vi "Draw Horizontal Line.vi"(6 "Colour":u32(colorbox), 9 "Point 2":T1, 10 "Point 1":T1, 11 "Pixel Data in":u32[][](array[numeric])) -> (3 "Pixel Data out":u32[][](array[numeric]))   [LabVIEW 2022 SP3, in "Raster.lvlib"]
uses:
  Raster.lvlib
  Point 2D.ctl
  <vilib>/Utility/High Resolution Relative Seconds.vi
  Utility/Utility.lvlib
panel:
  out "Processing Time [s]":dbl format="%.1p"
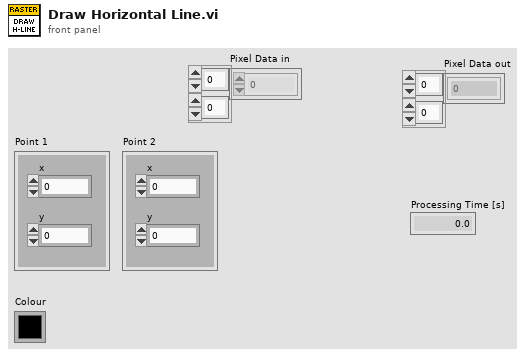
[diagram p1: front panel]
types:
  T1 = typedef "Raster.lvlib/Point 2D.ctl" = cluster{"x":i32, "y":i32}
  T2 = cluster{"pointer":u64, "size_0":u32, "stride_0":i32, "size_1":u32, "stride_1":i32, "element size":u32, "subarray?":bool}
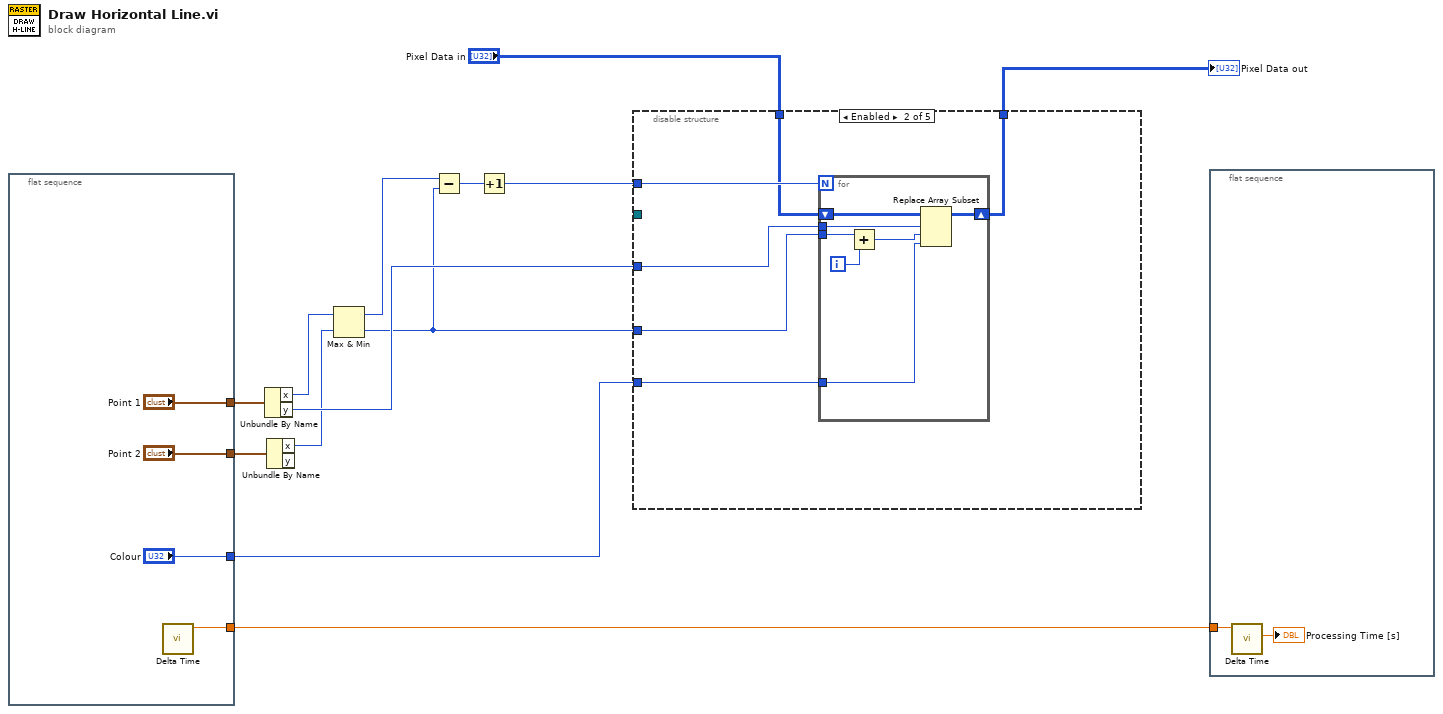
[diagram p0: block diagram]
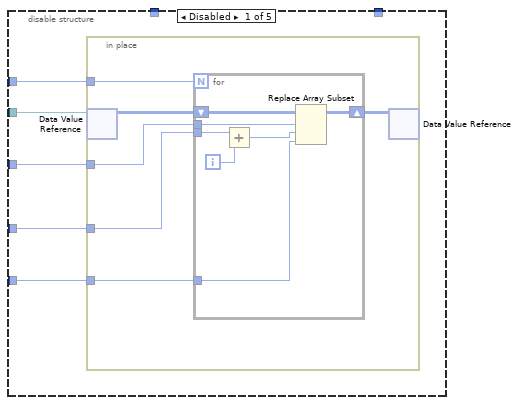
[diagram p2: hidden frame]
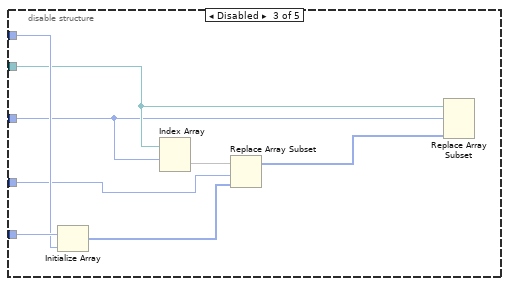
[diagram p3: hidden frame]
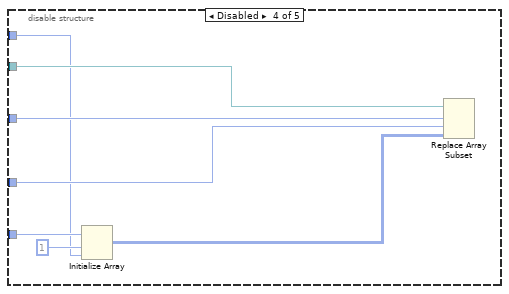
[diagram p4: hidden frame]
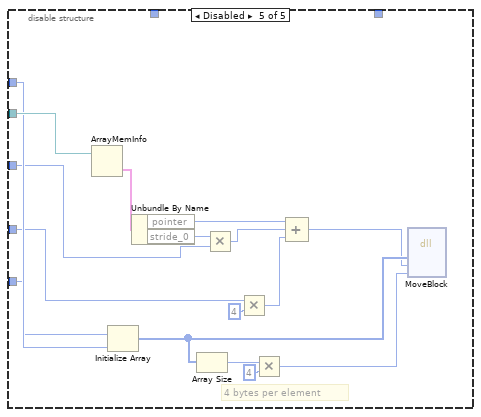
[diagram p5: hidden frame]
diagram:
  n1 = flat-sequence {
    tunnel: ["Point 1"] -> w12
    tunnel: ["Point 2"] -> w11
    tunnel: ["Colour"] -> w7
    tunnel: [w14] -> w13
    frame #0 {
      n2 = call "Delta Time.vi"() -> ("Relative Seconds Out"=w14:dbl)  [unwired: 10 in, 1 out]
    }
  }
  n3 = Unbundle By Name(w12) -> ("x"=w4:i32, "y"=w9:i32)
  n4 = Unbundle By Name(w11) -> ("x"=w6:i32)  [unwired: 1 out]
  n5 = Max & Min(x=w4, y=w6) -> (max(x,y)=w5:i32, min(x,y)=w3:i32)
  n6 = Subtract(x=w5, y=w3) -> (x-y=w10:i32)
  n7 = Increment(x=w10) -> (x+1=w8:i32)
  n8 = disable-structure shown="Enabled" {
    disable-tunnel: _ -> [w18 _ w54 w63 w79]
    disable-tunnel: w9 -> [w22 w41 w50 w62 w71]
    disable-tunnel: w8 -> [w21 w40 w55 w58 w78]
    disable-tunnel: w7 -> [w20 w39 w56 w64 w77]
    disable-tunnel: w3 -> [w19 w38 w51 w61 w68]
    disable-tunnel: "Pixel Data in" -> [_ w37 _ _ _]
    disable-tunnel: [_ w36 _ _ _] -> w1
    frame Disabled {
      n9 = in-place {
        in-place-border: w22 -> [w28]
        in-place-border: w21 -> [w27]
        in-place-border: w20 -> [w26]
        in-place-border: w19 -> [w25]
        n10 = in-place-dvr #1(w18) -> (w24:u32[][])  [unwired: 1 out]
        n11 = for {
          N: w27 -> [_]
          tunnel: w25 -> [w32]
          tunnel: w28 -> [w30]
          shift-right: [w34] -> w23
          shift-left: w24 -> [w35]
          tunnel: w26 -> [w29]
          i -> [w31]
          n12 = Add(x=w32, y=w31) -> (x+y=w33:i32)
          n13 = Replace Array Subset(array=w35, new element=w29, index (row)=w30, index (col)=w33) -> (w34:u32[][])
        }
        n14 = in-place-dvr #1(w23) -> ()  [unwired: 2 out]
      }
    }
    frame Enabled {
      n15 = for {
        N: w40 -> [_]
        tunnel: w38 -> [w45]
        tunnel: w41 -> [w43]
        shift-right: [w47] -> w36
        shift-left: w37 -> [w48]
        tunnel: w39 -> [w42]
        i -> [w44]
        n16 = Add(x=w45, y=w44) -> (x+y=w46:i32)
        n17 = Replace Array Subset(array=w48, new element=w42, index (row)=w43, index (col)=w46) -> (w47:u32[][])
      }
    }
    frame Disabled {
      n18 = Initialize Array(w56, w55) -> (w52:u32[])
      n19 = Index Array(array=w54, index (row)=w50) -> (element=w53)  [unwired: 1 in]
      n20 = Replace Array Subset(array=w53, new element=w52, index=w51) -> (w49:u32[])
      n21 = Replace Array Subset(array=w54, new element=w49, index (row)=w50) -> (w57:u32[])  [unwired: 1 in]
    }
    frame Disabled {
      n22 = Initialize Array(w64, 1 ("dimension size"), w58) -> (w60:u32[][])
      n23 = Replace Array Subset(array=w63, new element=w60, index (row)=w62, index (col)=w61) -> (w65:u32[])
    }
    frame Disabled {
      # "4 bytes per element"
      n24 = ArrayMemInfo(3:w79) -> (0:w81:T2, 1:w80:u32[][])
      n25 = Initialize Array(w77, w78) -> (w76:u32[])
      n26 = Unbundle By Name(w81) -> ("pointer"=w82:u64, "stride_0"=w72:i32)
      n27 = Array Size(array=w76) -> (size(s)=w75:i32)
      n28 = Multiply(x=w72, y=w71) -> (x*y=w70:i32)
      n29 = Multiply(x=w68, y=4) -> (x*y=w67:i32)
      n30 = Multiply(x=w75, y=4) -> (x*y=w73:i32)
      n31 = Compound Arithmetic op=ADD(w82, w70, w67) -> (w66:u64)
      n32 = dll-call lib="LabVIEW" fn="MoveBlock"("Src"=w76, "Dst"=w66, "Size"=w73) -> ()  [unwired: 7 in, 2 out]
    }
  }
  "Pixel Data out" <- w1
  n33 = flat-sequence {
    tunnel: w13 -> [w84]
    frame #0 {
      n34 = call "Delta Time.vi"("Relative Seconds In"=w84) -> ("Delta Time [s]"=→"Processing Time [s]":dbl)  [unwired: 9 in, 1 out]
    }
  }
